vi "Version Text to Number.vi"(11 "VersionText":string) -> (3 "Version Number":T1)   [LabVIEW 2016, in "Packages.lvlib"]
uses:
  Packages.lvlib
  Version Number--cluster.ctl
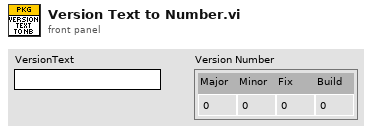
[diagram p1: front panel]
types:
  T1 = typedef "Packages.lvlib/Version Number--cluster.ctl" = cluster{"Major":i32, "Minor":i32, "Fix":i32, "Build":i32}
  T2 = cluster{"[0]":i32, "[1]":i32, "[2]":i32, "[3]":i32}
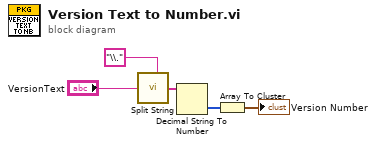
[diagram p0: block diagram]
diagram:
  n1 = call <vilib>:"Split String.vi"("Split Pattern"="\\.", "Input String"="VersionText") -> ("Split String"=w3:string[])  [unwired: 5 in]
  n2 = Decimal String To Number(string=w3) -> (number=w2:i32[])  [unwired: 2 in, 1 out]
  n3 = Array To Cluster(array=w2) -> (cluster=→"Version Number":T2)
